vi "Send Trigger.vi"(7 "Function":i32(ring) items=["DCI", "DCV"], 8 "error in (no error)":errorcluster, 11 "Digtal Multimeter in":refnum<class "Digital Multimeter.lvclass">) -> (0 "error out":errorcluster, 3 "Digtal Multimeter out":refnum<class "Digital Multimeter.lvclass">)   [LabVIEW 2020, in "Digital Multimeter.lvclass"]
uses:
  Digital Multimeter.lvclass
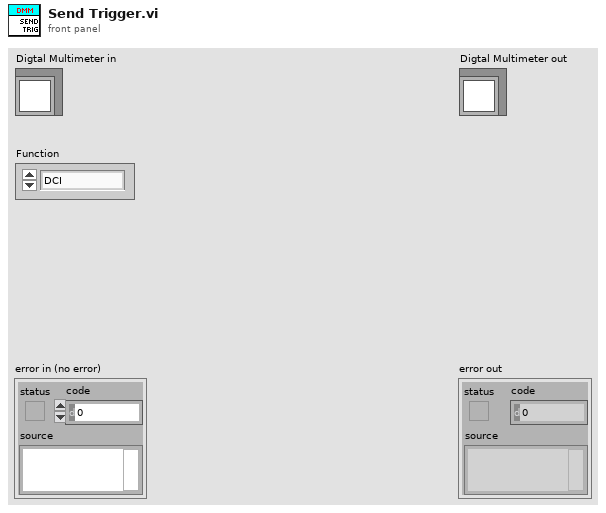
[diagram p1: front panel]
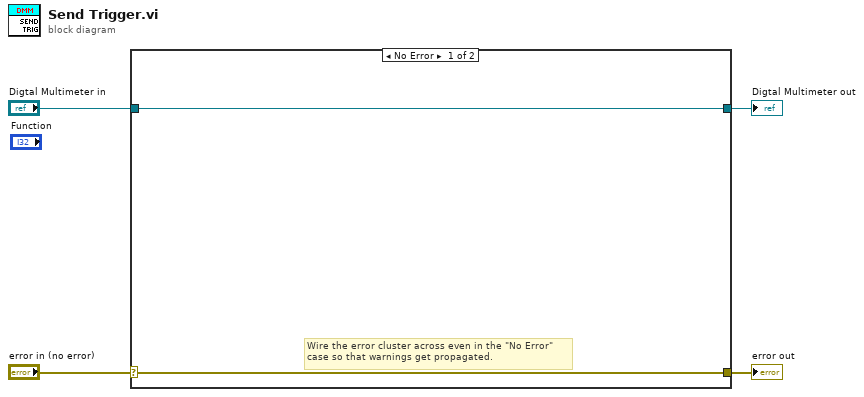
[diagram p0: block diagram]
diagram:
  n1 = case shown="No Error" "error in (no error)" {
    selector: "error in (no error)" -> [w5 w8]
    tunnel: [w5 w8] -> w3
    tunnel: [w6 w7] -> w1
    tunnel: "Digtal Multimeter in" -> [w6 w7]
    frame No Error {
      # "Wire the error cluster across even in the \"No Error\"\ncase so that warnings get propagated."
    }
    frame Error {
    }
  }
  "error out" <- w3
  "Digtal Multimeter out" <- w1
